vi "Modbus Sub.vi"() -> ()   [LabVIEW 2018]
uses:
  Temperature.lvlib
panel:
  out "Updating":bool
  in  "Update rate":dbl
  out "Off Hook":bool
  out "Communication Error":bool
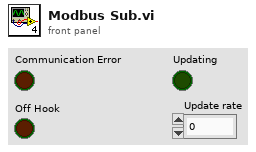
[diagram p1: front panel]
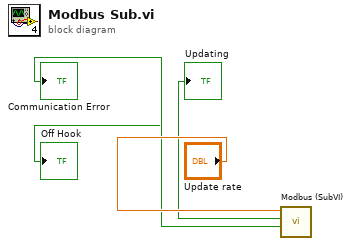
[diagram p0: block diagram]
diagram:
  n1 = call "Modbus (SubVI).vi"("Update rate"="Update rate") -> ("Off Hook"=→"Off Hook":bool, "Updating"=→"Updating":bool, "Communication Error"=→"Communication Error":bool)  [unwired: 8 in]
